vi "Select Moneda.vi"(10 "Moneda":i32, 11 "Credito":i32) -> (3 "New Credit":i32)   [LabVIEW 2020, in "Dinero.lvlib"]
uses:
  Dinero.lvlib
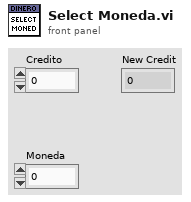
[diagram p1: front panel]
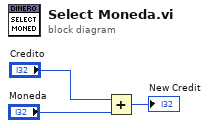
[diagram p0: block diagram]
diagram:
  n1 = Add(x="Credito", y="Moneda") -> (x+y=→"New Credit":i32)
